vi "LWXPS_PositionerCorrectorPIDBaseGet.vi"(0 "XPS Reference IN":refnum<k24>, 2 "Positioner Name":string, 5 "LabVIEW error IN":errorcluster) -> (12 "XPS Reference OUT":refnum<k24>, 13 "LabVIEW error OUT":errorcluster, 14 "Returned error code":i32, 15 "Moving Mass":dbl, 16 "Static Mass":dbl, 17 "Viscosity":dbl, 18 "Stiffness":dbl, 19 "XPS Error String":string)   [LabVIEW 2014]
uses:
  D:/XPSQ8_LabView_Library/Development/Source/Dll/Newport.XPS.CommandInterface.dll
  Dll/Newport.XPS.CommandInterface.dll
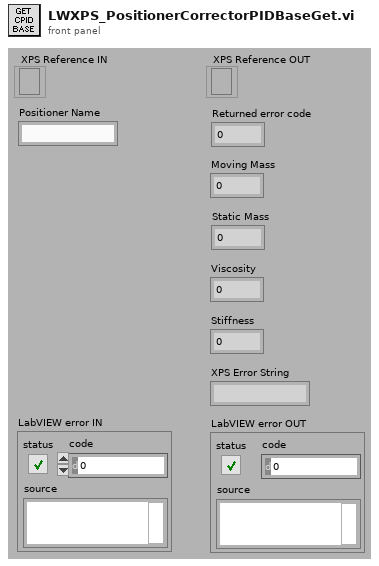
[diagram p1: front panel]
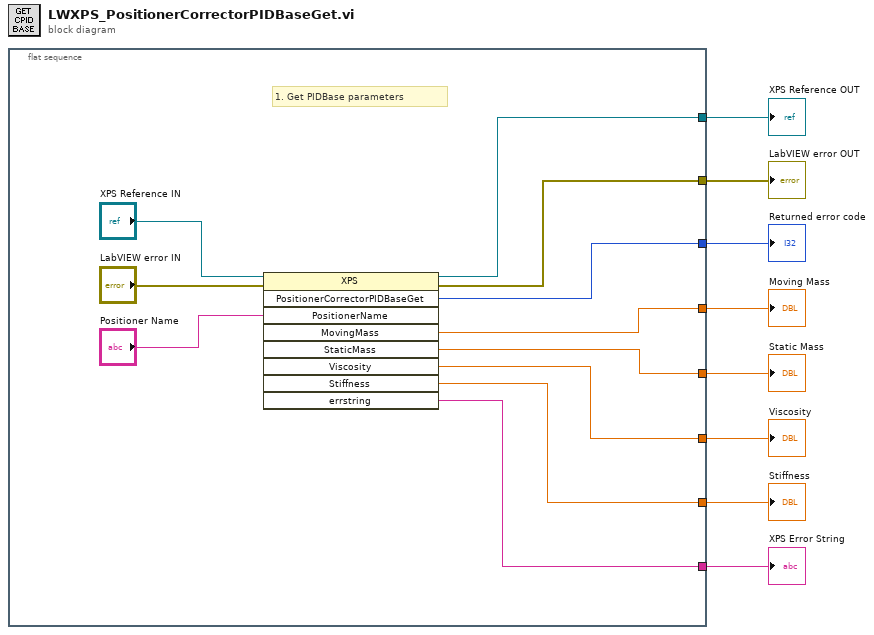
[diagram p0: block diagram]
diagram:
  n1 = flat-sequence {
    tunnel: [w17] -> w8
    tunnel: [w14] -> w7
    tunnel: [w18] -> w6
    tunnel: [w12] -> w4
    tunnel: [w13] -> w5
    tunnel: [w10] -> w1
    tunnel: [w11] -> w3
    tunnel: [w9] -> w2
    frame #0 {
      # "1. Get PIDBase parameters"
      n2 = invoke class="XPS" method="PositionerCorrectorPIDBaseGet"(reference="XPS Reference IN", error in="LabVIEW error IN", "PositionerName"="Positioner Name") -> (reference out=w17:refnum<k24>, error out=w14:errorcluster, "PositionerCorrectorPIDBaseGet"=w18:i32, "MovingMass"=w12:dbl, "StaticMass"=w13:dbl, "Viscosity"=w11:dbl, "Stiffness"=w10:dbl, "errstring"=w9:string)  [unwired: 6 in, 1 out]
    }
  }
  "XPS Error String" <- w2
  "XPS Reference OUT" <- w8
  "LabVIEW error OUT" <- w7
  "Returned error code" <- w6
  "Static Mass" <- w5
  "Moving Mass" <- w4
  "Viscosity" <- w3
  "Stiffness" <- w1
